vi "Get_Set_Status_id.vi"(6 "Get/Set":T1, 8 "Status/Errors in":refnum<vi>, 9 "Status_id":refnum<vi>, 11 "Value in":u8) -> (0 "Status/Errors out":refnum<vi>, 1 "Status_out":refnum<vi>, 3 "Value out":u8)   [LabVIEW 2010]
uses:
  Controls/Get_Set_Statistics_Options2.ctl
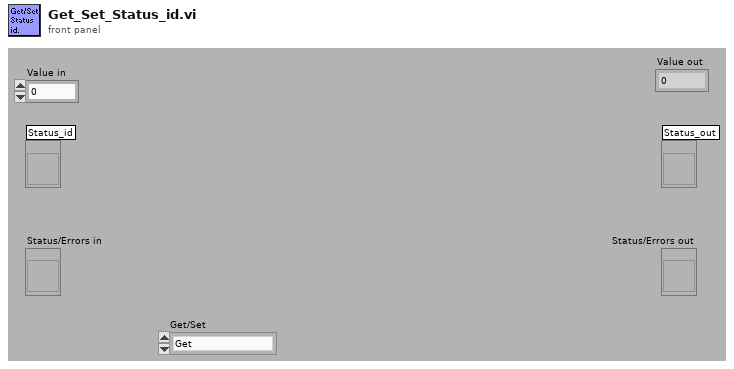
[diagram p1: front panel]
types:
  T1 = typedef "Get_Set_Statistics_Options2.ctl" = enum16{"Get", "Set"}
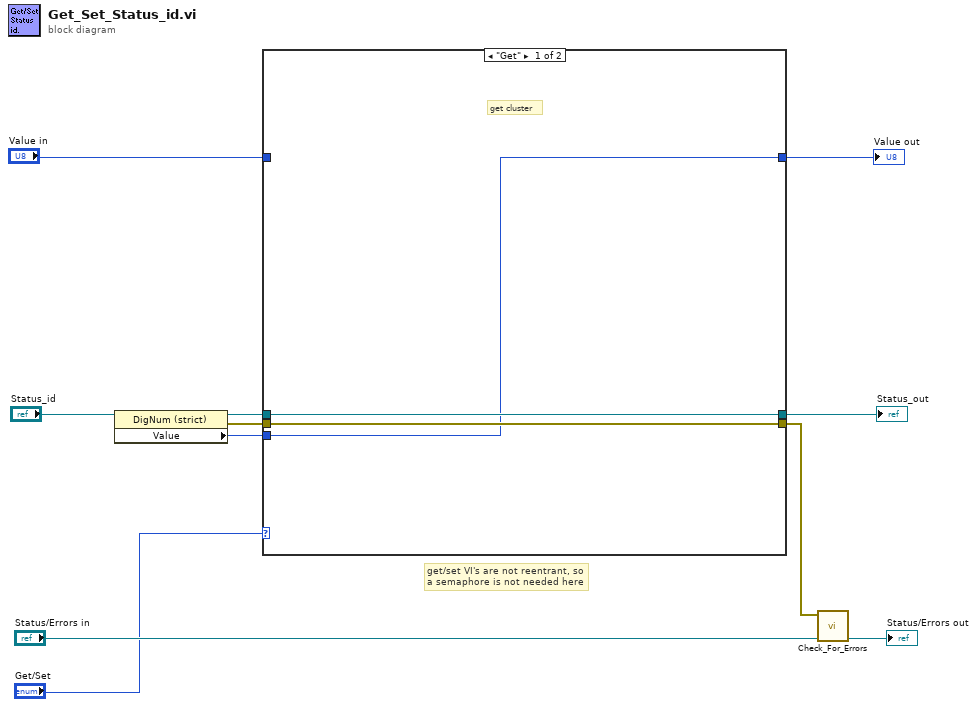
[diagram p0: block diagram]
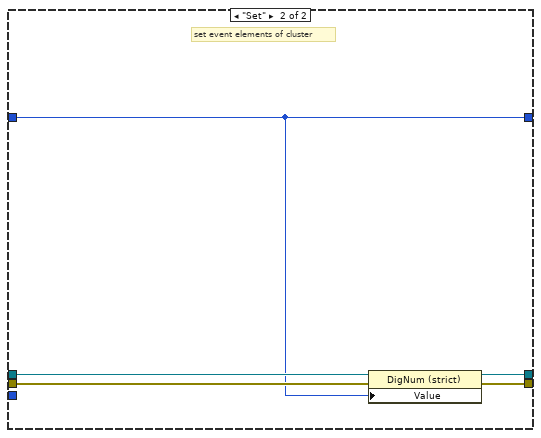
[diagram p2: hidden frame]
diagram:
  # "get/set VI's are not reentrant, so\na semaphore is not needed here"
  n1 = property class="DigNum (strict)"(reference="Status_id") -> (reference out=w7:refnum<vi>, error out=w8:errorcluster, "Value"=w6:u8)  [unwired: 1 in]
  n2 = case shown="\"Get\"" "Get/Set" {
    tunnel: "Value in" -> [_ w15]
    tunnel: w7 -> [w14 w16]
    tunnel: [w14 w18] -> w1
    tunnel: [w13 w19] -> w10
    tunnel: w6 -> [w12 _]
    tunnel: w8 -> [w13 w17]
    tunnel: [w12 w15] -> w2
    frame "Get" {
      # "get cluster"
    }
    frame "Set" {
      # "set event elements of cluster"
      n3 = property class="DigNum (strict)"(reference=w16, error in=w17, "Value"=w15) -> (reference out=w18:refnum<vi>, error out=w19:errorcluster)
    }
  }
  "Value out" <- w2
  "Status_out" <- w1
  n4 = call "Check_For_Errors.vi"("Status/Errors in"="Status/Errors in", "error in"=w10) -> ("Status/Errors out"=→"Status/Errors out":refnum<vi>)  [unwired: 9 out]
